vi "RGB FFT.vi"(8 "New Value":u32, 9 "Array In":i32[](array[numeric])) -> (0 "error out":errorcluster, 1 "Array Out":i32[](array[numeric]), 3 "Magnitude Array":dbl[](array[numeric]), 4 "R FFT":dbl[](graph), 6 "R Input":dbl[](graph))   [LabVIEW 2019]
uses:
  <vilib>/Analysis/2dsp.llb/Real FFT.vi
  <vilib>/Analysis/NI_AALPro.lvlib
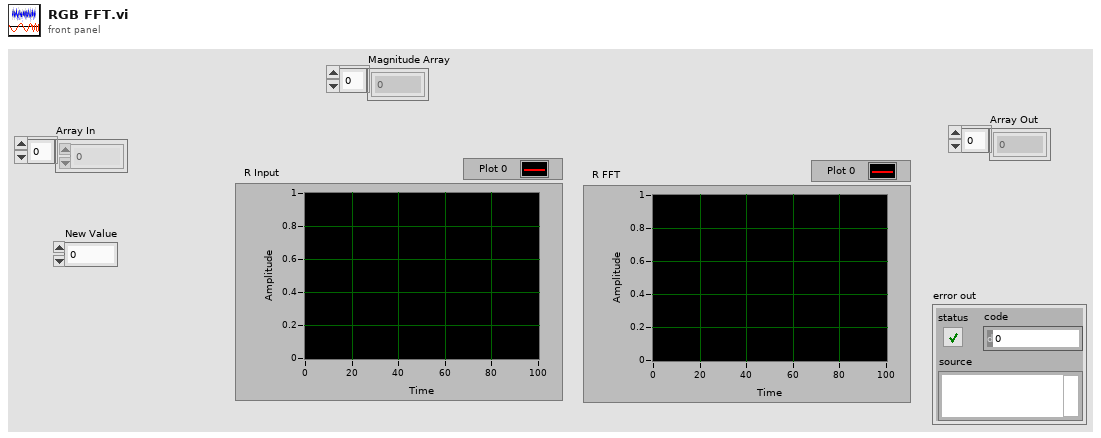
[diagram p1: front panel]
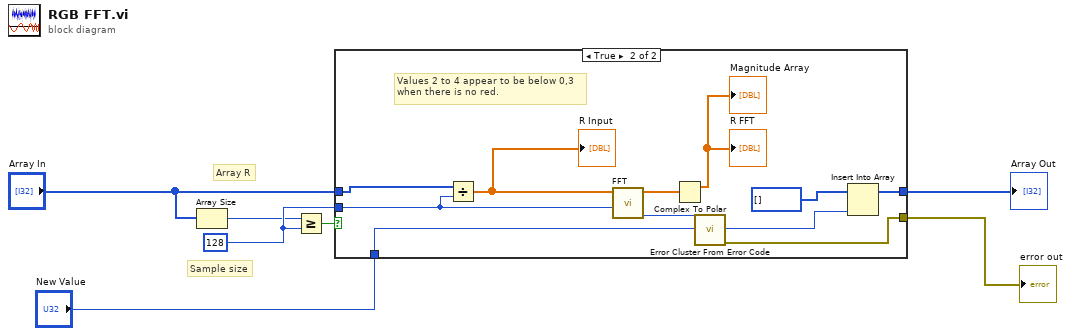
[diagram p0: block diagram]
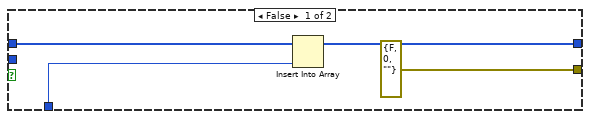
[diagram p2: hidden frame]
diagram:
  w6 = 128
  # "Array R"
  # "Sample size"
  n1 = Array Size(array="Array In") -> (size(s)=w4:i32)
  n2 = Greater Or Equal?(x=w4, y=w6) -> (x >= y?=w7:bool)
  n3 = case shown="True" w7 {
    tunnel: "Array In" -> [w10 w16]
    tunnel: "New Value" -> [w11 w18]
    tunnel: [w9 w19] -> w3
    tunnel: [errorcluster {"status"=FALSE, "code"=0, "source"=""} ("error constant") w12] -> w5
    tunnel: w6 -> [_ w15]
    frame False {
      n4 = Insert Into Array(array=w10, new element=w11) -> (w9:i32[])  [unwired: 1 in]
    }
    frame True {
      # "Values 2 to 4 appear to be below 0,3\nwhen there is no red."
      n5 = Divide(x=w16, y=w15) -> (x/y=w13:dbl[])
      "R Input" <- w13
      n6 = call-poly <vilib>:"FFT.vi"("FFT size"=w15, "X"=w13) -> ("error"=w17:i32, "FFT {X}"=w21:cdb[])  [unwired: 8 in]
      n7 = Complex To Polar(r * e^(i*theta)=w21) -> (r=→"R FFT" →"Magnitude Array":dbl[])  [unwired: 1 out]
      n8 = call <vilib>:"Error Cluster From Error Code.vi"("error code (0)"=w17) -> ("error out"=w12:errorcluster)  [unwired: 8 in]
      n9 = Insert Into Array(array=i32[] [], new element=w18) -> (w19:i32[])  [unwired: 1 in]
    }
  }
  "Array Out" <- w3
  "error out" <- w5
